vi "Cast Request.vi"(11 "Client Message":refnum<class "Client Message.lvclass">) -> (2 "Is Request?":bool, 3 "Request":refnum<class "Request.lvclass">)   [LabVIEW 2022 SP3, in "obs-websocket-lv.lvlib"]
uses:
  obs-websocket-lv.lvlib
  Client Message/Client Message.lvclass
  Request/Request.lvclass
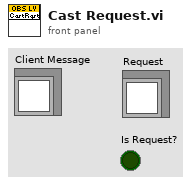
[diagram p1: front panel]
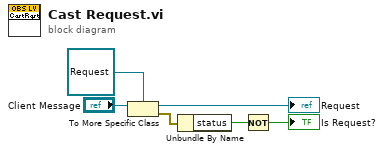
[diagram p0: block diagram]
diagram:
  n1 = To More Specific Class(target class=refnum<class "Request.lvclass"> refnum ("Request"), reference="Client Message") -> (specific class reference=→"Request":refnum<class "Request.lvclass">, error out=w3:errorcluster)  [unwired: 1 in]
  n2 = Unbundle By Name(w3) -> ("status"=w2:bool)
  n3 = Not(x=w2) -> (.not. x?=→"Is Request?":bool)
